vi "Generate-CMD-Datastruct.vi"() -> ()   [LabVIEW 2020, in "Generate-Go-CMD.lvlib"]
uses:
  Generate-Go-CMD.lvlib
  <vilib>/Utility/Data Type/NI_Data Type.lvlib
panel:
  in  "CMD":variant
  out "error out":errorcluster
  in  "error in (no error)":errorcluster
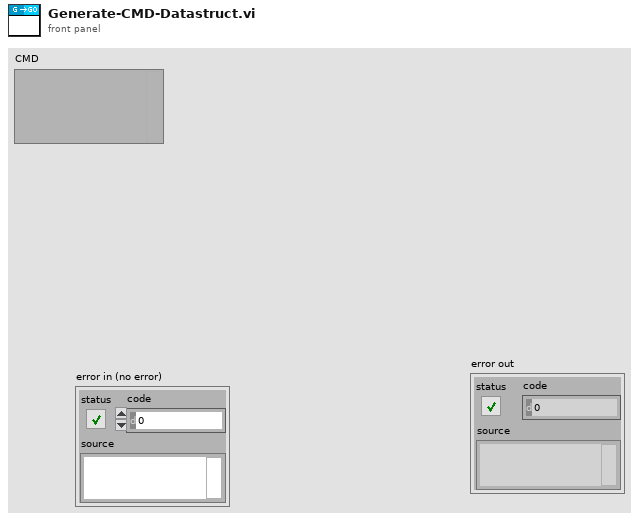
[diagram p1: front panel]
types:
  T1 = typedef "NI_Data Type.lvlib/Data Type.ctl" = enum8{"Invalid Type", "Void", "I8", "I16", "I32", "I64", "U8", "U16", "U32", "U64", "Single Float", "Double Float", "Extended Float", "Single Complex", "Double Complex", "Extended Complex", "Enum U8", "Enum U16", "Enum U32", "Enum U64", "Single Float With Unit", "Double Float With Unit", "Extended Float With Unit", "Single Complex with Unit", "Double Complex with Unit", "Extended Complex with Unit", "Boolean", "String", "Path", "Picture", "Tag", "Array", "Cluster", "Variant", "LV Variant", "Waveform", "Timestamp", "Digital Waveform", "Digital Data", "ExpressData", "Refnum", "External Data", "VI", "Poly VI", "LabVIEW Class Instance", "Fixed Point", "Set Collection", "Map Collection"}
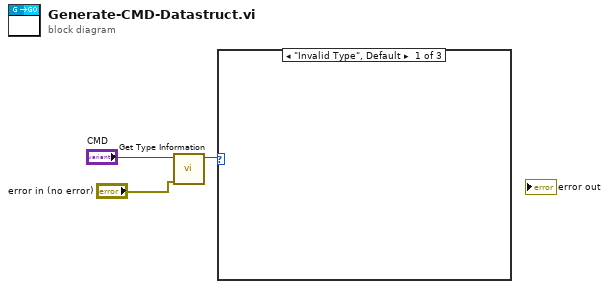
[diagram p0: block diagram]
diagram:
  n1 = call <vilib>:"Get Type Information.vi"("error in (no error)"="error in (no error)", "variant"="CMD") -> ("type"=w1:T1)  [unwired: 5 in, 4 out]
  n2 = case shown="\"Invalid Type\", Default" w1 {
    frame "Invalid Type", Default {
    }
    frame "Void" {
    }
    frame "I8" {
    }
  }
